vi "Get Name.vi"(7 "Unique ID":string, 8 "error in (no error)":errorcluster, 11 "Test Executive Ref":refnum<data-value>) -> (0 "error out":errorcluster, 1 "Tag":i32, 2 "Name":string, 3 "Test Executive Ref out":refnum<data-value>, 4 "Class":string)   [LabVIEW 2020, in "Test Executive.lvlib" / "TestExecutive Ref.lvclass"]
uses:
  <vilib>/gpm_packages/@cs/test-executive/Source/Test Executive/TestExecutive Ref/TestExecutive Ref.lvclass
  <vilib>/gpm_packages/@cs/test-executive/Source/Test Executive/ITestExecutive/ITest Executive.lvclass
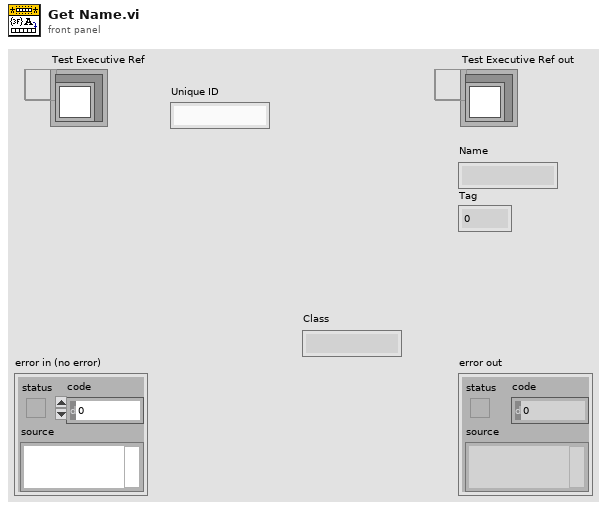
[diagram p1: front panel]
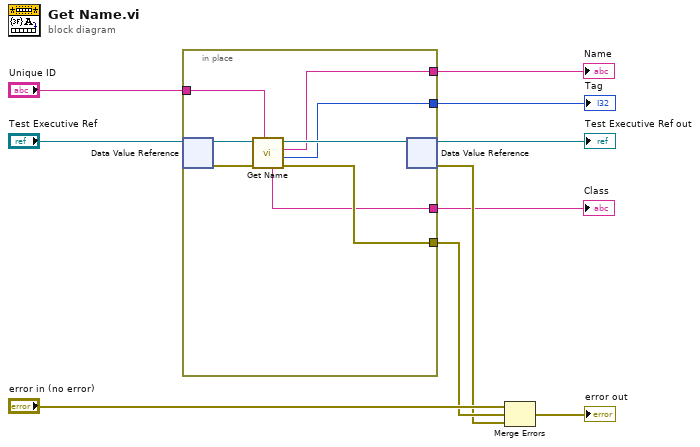
[diagram p0: block diagram]
diagram:
  n1 = in-place {
    in-place-border: "Unique ID" -> [w18]
    in-place-border: [w14] -> w6
    in-place-border: [w13] -> w3
    in-place-border: [w12] -> w2
    in-place-border: [w11] -> w1
    n2 = in-place-dvr #1("Test Executive Ref") -> (w17:refnum<class "ITest Executive.lvclass">, w15:errorcluster)
    n3 = call-dynamic "Get Name.vi"("Unique ID"=w18, "error in (no error)"=w15, "ITest Executive in"=w17) -> ("error out"=w14:errorcluster, "Tag"=w12:i32, "Name"=w13:string, "ITest Executive out"=w16:refnum<class "ITest Executive.lvclass">, "Class"=w11:string)  [unwired: 4 in]
    n4 = in-place-dvr #1(w16) -> (→"Test Executive Ref out":refnum<data-value>, w5:errorcluster)
  }
  "Name" <- w3
  "Tag" <- w2
  "Class" <- w1
  n5 = Merge Errors("error in (no error)", w6, w5) -> (→"error out":errorcluster)
